vi "Timing Engine Unit Test Main.vi"(8 "Ramp Data Array":T1[](array[typedef]), 9 "Ramp?":bool, 10 "Length of Test":u32=10000, 11 "Starting Timer Rate":i32=100) -> (3 "Return Value":i32)   [LabVIEW 2017, in "Timing Engine Tester.lvlib"]
uses:
  Timing Engine Tester.lvlib
  Timing Engine Tester/Ramp Data.ctl
  Timing Engine Tester/Timing Engine Tester.lvclass
  C:/Program Files (x86)/National Instruments/LabVIEW 2017/vi.lib/ActorFramework/Actor/Actor.lvclass
  Timing Engine Tester/Timing Engine Tester.lvclass/Timing Engine Tester.ctl
  Timing Engine Tester Messages/Update Test Timer Msg/Update Test Timer Msg.lvclass/Update Test Timer Msg.ctl
  <vilib>/ActorFramework/Message Enqueuer/Message Enqueuer.lvclass/Message Enqueuer.ctl
  <vilib>/ActorFramework/Message Enqueuer/Enqueue.vi
  Timing Engine Tester Messages/Update Test Timer Msg/Update Test Timer Msg.lvclass
  C:/Program Files (x86)/National Instruments/LabVIEW 2017/vi.lib/ActorFramework/Message/Message.lvclass
  <vilib>/ActorFramework/Stop Msg/Stop Msg.lvclass
  <vilib>/Utility/LVClass/Get LV Class Name.vi
  <resource>/AFDebug/Generate Trace for Message.vi
  <vilib>/ActorFramework/Message Priority Queue/Priority Enqueue.vi
  <vilib>/ActorFramework/Actor/Actor.lvclass
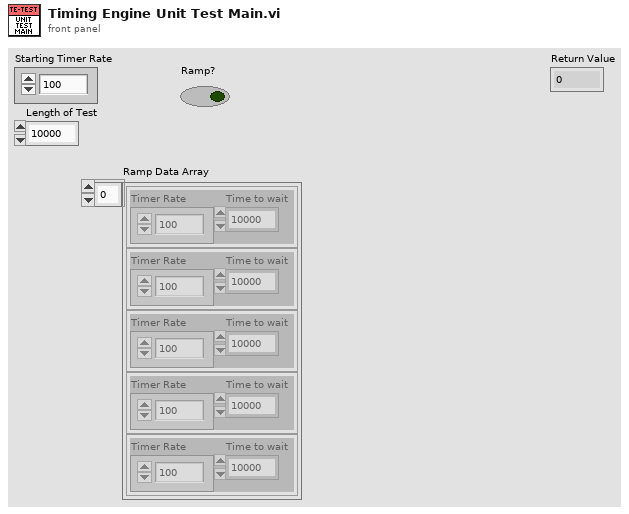
[diagram p1: front panel]
types:
  T1 = typedef "Timing Engine Tester.lvlib/Ramp Data.ctl" = cluster{"Timer Rate":i32, "Time to wait":u32}
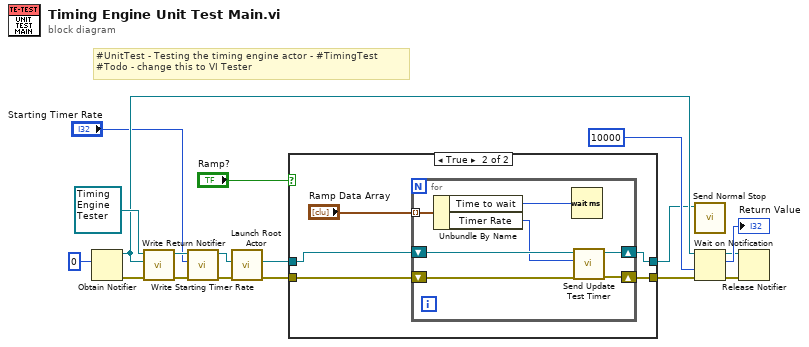
[diagram p0: block diagram]
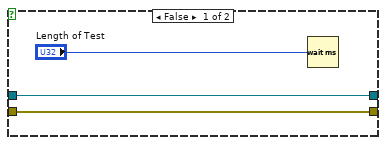
[diagram p2: hidden frame]
diagram:
  # "#UnitTest - Testing the timing engine actor - #TimingTest\n#Todo - change this to VI Tester"
  n1 = Obtain Notifier(notification data type=0) -> (notifier out=w16:refnum<notifier>, error out=w6:errorcluster)  [unwired: 3 in, 1 out]
  n2 = call "Write Return Notifier.vi"("error in (no error)"=w6, "Return Notifier"=w16, "Timing Engine Tester in"=refnum<class "Timing Engine Tester.lvclass"> refnum ("Assert API Components.lvlib:Assert Display.lvlib:Timing Engine Tester.lvlib:Timing Engine Tester.lvclass")) -> ("error out"=w8:errorcluster, "Timing Engine Tester out"=w11:refnum<class "Timing Engine Tester.lvclass">)  [unwired: 7 in]
  n3 = call "Write Starting Timer Rate.vi"("error in (no error)"=w8, "Starting Timer Rate"="Starting Timer Rate", "Timing Engine Tester in"=w11) -> ("error out"=w9:errorcluster, "Timing Engine Tester out"=w10:refnum<class "Timing Engine Tester.lvclass">)  [unwired: 7 in]
  n4 = call <vilib>:"Launch Root Actor.vi"("error in (no error)"=w9, "Actor"=w10) -> ("error out"=w1:errorcluster, "Actor's Enqueuer"=w3:refnum<class "Message Enqueuer.lvclass">)  [unwired: 8 in]
  n5 = case shown="True" "Ramp?" {
    tunnel: [w20 w25] -> w4
    tunnel: w3 -> [w20 w26]
    tunnel: [w19 w22] -> w2
    tunnel: w1 -> [w19 w23]
    frame False {
      n6 = Wait (ms)(milliseconds to wait="Length of Test") -> ()  [unwired: 1 out]
    }
    frame True {
      n7 = for {
        shift-right: [w32] -> w25
        shift-left: w26 -> [w33]
        tunnel: "Ramp Data Array" -> [w31] mode=indexing
        shift-right: [w27] -> w22
        shift-left: w23 -> [w28]
        n8 = Unbundle By Name(w31) -> ("Time to wait"=w29:u32, "Timer Rate"=w30:i32)
        n9 = Wait (ms)(milliseconds to wait=w29) -> ()  [unwired: 1 out]
        n10 = call "Send Update Test Timer.vi"("error in (no error)"=w28, "Timeout Value"=w30, "Message Enqueuer"=w33) -> ("error out"=w27:errorcluster, "Message Enqueuer out"=w32:refnum<class "Message Enqueuer.lvclass">)  [unwired: 7 in]
      }
    }
  }
  n11 = call <vilib>:"Send Normal Stop.vi"("Message Enqueuer"=w4) -> ()  [unwired: 10 in, 1 out]
  n12 = Wait on Notification(notifier=w16, timeout in ms (-1)=10000, error in (no error)=w2) -> (notifier out=w13:refnum<notifier>, notification=→"Return Value":i32, error out=w12:errorcluster)  [unwired: 1 in, 1 out]
  n13 = Release Notifier(notifier=w13, error in (no error)=w12) -> ()  [unwired: 1 in, 3 out]
